vi "Configure Sweep Mode.vi"(8 "error in (no error)":errorcluster, 10 "Sweep Mode":enum16{"Continuous", "Single"}(ring), 11 "SA-FSW in":refnum<class "SA-FSW.lvclass">) -> (0 "error out":errorcluster, 3 "SA-FSW out":refnum<class "SA-FSW.lvclass">)   [LabVIEW 2020, in "SA-FSW.lvclass"]
uses:
  SA-FSW.lvclass
  C:/Sandbox/RF Bench/Source Code/WiSpry Test Framework/Instruments/Instrument.lvclass
  Instrument.lvclass/Instrument.ctl
  Instrument.lvclass
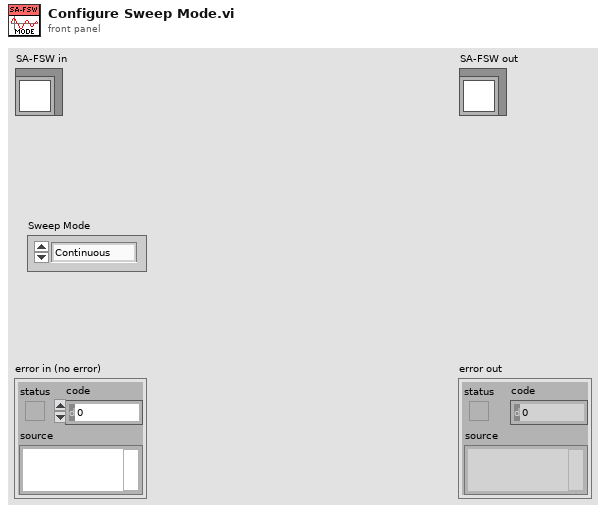
[diagram p1: front panel]
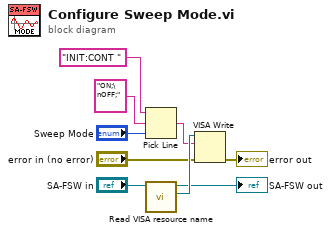
[diagram p0: block diagram]
diagram:
  n1 = Pick Line(string ("")="INIT:CONT ", multi-line string="ON;\nOFF;", line index="Sweep Mode") -> (output string=w4:string)
  n2 = call "Read VISA resource name.vi"("Instrument in"="SA-FSW in") -> ("VISA resource name"=w5:refnum<visa-resource-name>, "Instrument out"=→"SA-FSW out":refnum<class "SA-FSW.lvclass">)  [unwired: 9 in]
  n3 = VISA Write(VISA resource name=w5, write buffer=w4, error in (no error)="error in (no error)") -> (error out=→"error out":errorcluster)  [unwired: 2 out]
